vi "set_new_position.vi"(8 "error in (no error)":errorcluster, 10 "set_pos":dbl[](array[numeric]), 11 "dummyStageRapid in":refnum<class "dummyStageRapid.lvclass">) -> (0 "error out":errorcluster, 3 "dummyStageRapid out":refnum<class "dummyStageRapid.lvclass">)   [LabVIEW 2019, in "dummyStageRapid.lvlib" / "dummyStageRapid.lvclass"]
uses:
  dummyStageRapid.lvclass
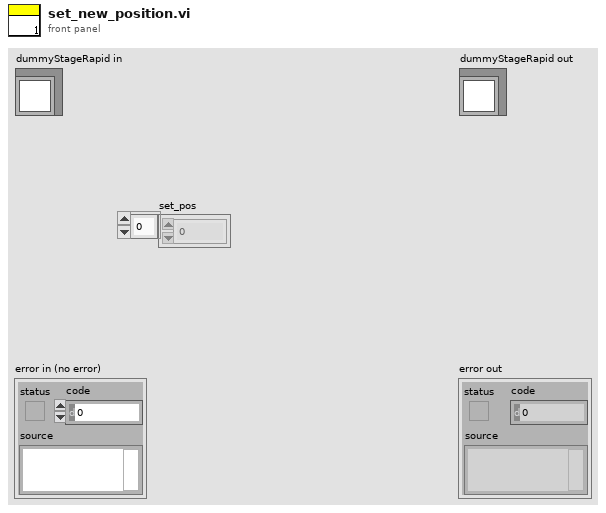
[diagram p1: front panel]
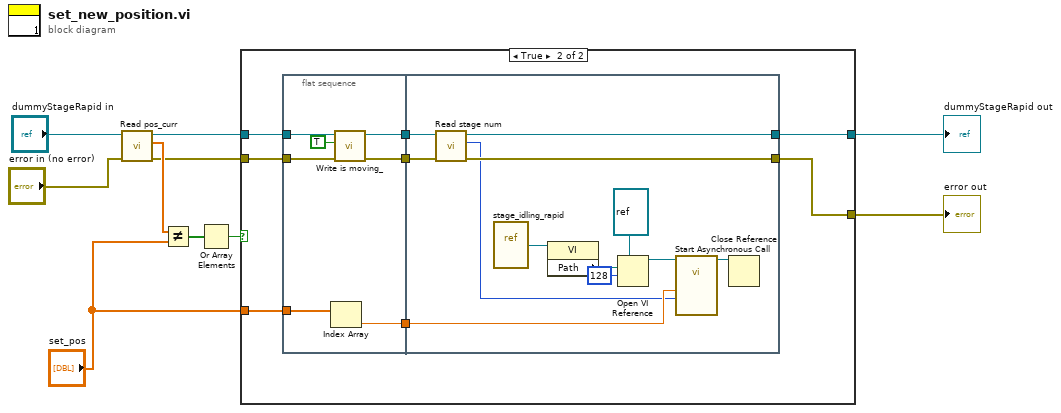
[diagram p0: block diagram]
diagram:
  n1 = call-dynamic "Read pos_curr.vi"("error in (no error)"="error in (no error)", "_stage in"="dummyStageRapid in") -> ("error out"=w5:errorcluster, "readback position"=w7:dbl[], "_stage out"=w4:refnum<class "dummyStageRapid.lvclass">)  [unwired: 7 in]
  n2 = Not Equal?(x=w7, y="set_pos") -> (x != y?=w8:bool[])
  n3 = Or Array Elements(Boolean array=w8) -> (logical OR=w6:bool)
  n4 = case shown="True" w6 {
    tunnel: w5 -> [w11 w19]
    tunnel: w4 -> [w12 w20]
    tunnel: [w11 w16] -> w3
    tunnel: "set_pos" -> [_ w15]
    tunnel: [w12 w13] -> w1
    frame False {
    }
    frame True {
      n5 = flat-sequence {
        tunnel: w20 -> [w27]
        tunnel: w19 -> [w26]
        tunnel: [w25] -> w18
        tunnel: [w24] -> w17
        tunnel: w15 -> [w23]
        tunnel: [w22] -> w14
        tunnel: w18 -> [w39]
        tunnel: w17 -> [w38]
        tunnel: [w37] -> w13
        tunnel: [w36] -> w16
        tunnel: w14 -> [w29]
        frame #0 {
          n6 = Index Array(array=w23) -> (element=w22:dbl)  [unwired: 1 in]
          n7 = call-dynamic "Write is moving_.vi"("error in (no error)"=w26, "is moving?"=TRUE, "_stage in"=w27) -> ("error out"=w24:errorcluster, "_stage out"=w25:refnum<class "dummyStageRapid.lvclass">)  [unwired: 7 in]
        }
        frame #1 {
          n8 = call-dynamic "Read stage num.vi"("error in (no error)"=w38, "_stage in"=w39) -> ("error out"=w36:errorcluster, "stage num"=w28:u8, "_stage out"=w37:refnum<class "dummyStageRapid.lvclass">)  [unwired: 7 in]
          n9 = vi-ref "stage_idling_rapid.vi"() -> (w31:refnum<vi>)
          n10 = property class="VI"(reference=w31) -> ("Path"=w34:path)  [unwired: 1 in, 2 out]
          n11 = Open VI Reference(type specifier VI Refnum (for type only)=refnum<vi> refnum, vi path=w34, options=128) -> (vi reference=w33:refnum<vi>)  [unwired: 3 in, 1 out]
          n12 = call-by-ref "Start Asynchronous Call"(reference=w33, "num"=w28, "pos"=w29) -> (reference out=w32:refnum<vi>)  [unwired: 11 in, 1 out]
          n13 = Close Reference(reference=w32) -> ()  [unwired: 1 in, 1 out]
        }
      }
    }
  }
  "error out" <- w3
  "dummyStageRapid out" <- w1
